vi "check_mouse_input_for_ROI.vi"() -> ()   [LabVIEW 2010]
uses:
  <vilib>/Utility/miscctls.llb/LVPoint32TypeDef.ctl
panel:
  in  "output cluster 2":T2
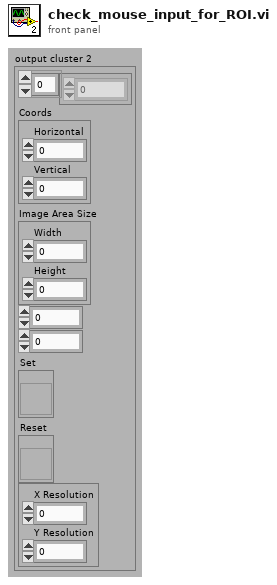
[diagram p1: front panel]
types:
  T1 = typedef "LVPoint32TypeDef.ctl" = cluster{"Horizontal":i32, "Vertical":i32}
  T2 = cluster{dbl[], "Coords":T1, "Image Area Size":cluster{"Width":u32, "Height":u32}, i32, i32, "Set":refnum<vi>, "Reset":refnum<vi>, cluster{"X Resolution":i32, "Y Resolution":i32}}
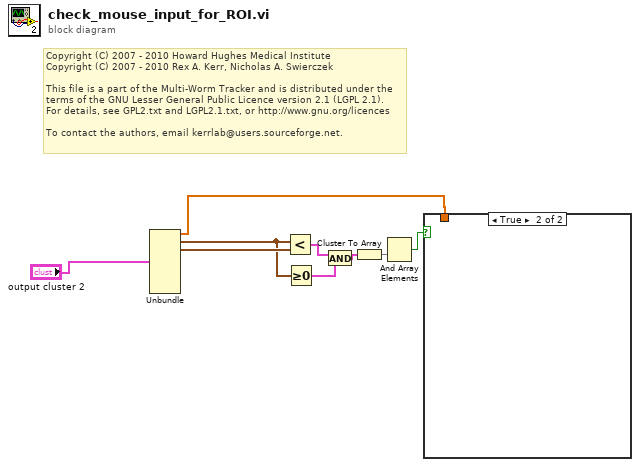
[diagram p0: block diagram]
diagram:
  # "Copyright (C) 2007 - 2010 Howard Hughes Medical Institute\nCopyright (C) 2007 - 2010 Rex A. Kerr, Nicholas A. Swierczek\n \nThis file is a part of the Multi-Worm Tracker and is distributed under the\nterms of the GNU Lesser General Public Licence version 2.1 (LGPL 2.1).\nFor details, see GPL2.txt and LGPL2.1.txt, or http://www.gnu.org/licences\n \nTo contact the authors, email kerrlab@users.sourceforge.net."
  n1 = Unbundle("output cluster 2") -> (w1:dbl[], "Coords"=w5:T1, "Image Area Size"=w8:cluster{"Width":u32, "Height":u32})  [unwired: 5 out]
  n2 = Less?(x=w5, y=w8) -> (x < y?=w7:cluster{bool, bool})
  n3 = Greater Or Equal To 0?(x=w5) -> (x >= 0?=w6:cluster{"Horizontal":bool, "Vertical":bool})
  n4 = And(x=w7, y=w6) -> (x .and. y?=w4:cluster{bool, bool})
  n5 = Cluster To Array(cluster=w4) -> (array=w3:bool[])
  n6 = And Array Elements(Boolean array=w3) -> (logical AND=w2:bool)
  n7 = case shown="True" w2 {
    tunnel: w1 -> [_ _]
    frame False {
    }
    frame True {
    }
  }
